vi "Keithley2400series_Start.vi"(4 "Serial Configuration":T1={"Baud Rate"=9600, "Parity"=0, "Data Bits"=8, "Stop Bits"=10, "Flow Control"=0} {"Flow Control" items=["None", "XON/XOFF", "RTS/CTS", "XON/XOFF & RTS/CTS", "DTR/DSR", "XON/XOFF & DTR/DSR"]; "Stop Bits" items=["1.0"=10, "1.5"=15, "2.0"=20]; "Data Bits" items=["7"=7, "8"=8]; "Parity" items=["None", "Odd", "Even", "Mark", "Space"]; "Baud Rate" items=["300"=300, "600"=600, "1200"=1200, "2400"=2400, "4800"=4800, "9600"=9600, "19200"=19200]}, 5 "Source Mode  (0: Voltage) 2":u16(ring) items=["Voltage", "Current"], 6 "Ограничение":dbl format="%.2f", 7 "Выход":dbl, 8 "VISA resource name":refnum<visa-resource-name>) -> (0 "error out":errorcluster, 1 "MEAS:Out":string, 2 "MEAS mode 0,Volt":dbl, 3 "VISA resource name out":refnum<visa-resource-name>)   [LabVIEW 2014]
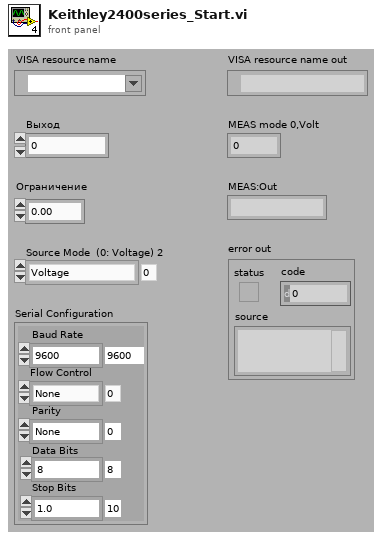
[diagram p1: front panel]
types:
  T1 = cluster{"Baud Rate":u32, "Parity":u16, "Data Bits":u16, "Stop Bits":u16, "Flow Control":u16}
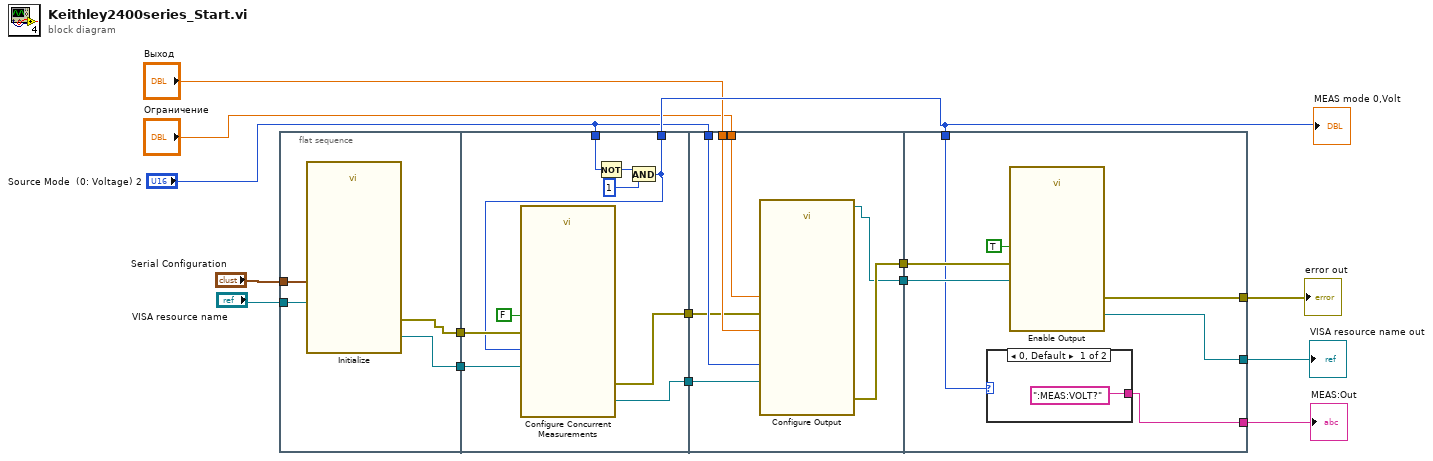
[diagram p0: block diagram]
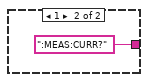
[diagram p2: hidden frame]
diagram:
  n1 = flat-sequence {
    tunnel: "VISA resource name" -> [w19]
    tunnel: "Serial Configuration" -> [w18]
    tunnel: [w17] -> w15
    tunnel: [w16] -> w14
    tunnel: "Source Mode  (0: Voltage) 2" -> [w25]
    tunnel: [w24] -> w13
    tunnel: [w23] -> w12
    tunnel: w15 -> [w22]
    tunnel: w14 -> [w21]
    tunnel: [w20] -> w9
    tunnel: "Ограничение" -> [w35]
    tunnel: "Выход" -> [w34]
    tunnel: "Source Mode  (0: Voltage) 2" -> [w33]
    tunnel: [w32] -> w11
    tunnel: [w31] -> w10
    tunnel: w13 -> [w30]
    tunnel: w12 -> [w29]
    tunnel: w11 -> [w41]
    tunnel: w10 -> [w40]
    tunnel: w9 -> [w39]
    tunnel: [w38] -> w5
    tunnel: [w37] -> w6
    tunnel: [w36] -> w7
    frame #0 {
      n2 = call "Initialize.vi"("Serial Configuration"=w18, "VISA resource name"=w19) -> ("error out"=w16:errorcluster, "VISA resource name out"=w17:refnum<visa-resource-name>)  [unwired: 8 in]
    }
    frame #1 {
      n3 = Not(x=w25) -> (.not. x?=w27:u16)
      n4 = And(x=w27, y=u16 1) -> (x .and. y?=w20:u16)
      n5 = call "Configure Concurrent Measurements.vi"("error in (no error)"=w21, "Measurement Selection (3: Volts, Current)"=w20, "Enable Concurrent Measurements (F: Disable)"=FALSE, "VISA resource name"=w22) -> ("error out"=w23:errorcluster, "VISA resource name out"=w24:refnum<visa-resource-name>)  [unwired: 6 in]
    }
    frame #2 {
      n6 = call "Configure Output.vi"("Source Mode  (0: Voltage)"=w33, "error in (no error)"=w29, "Compliance  Level (0.1)"=w35, "Output Level (0)"=w34, "VISA resource name"=w30) -> ("error out"=w32:errorcluster, "VISA resource name out"=w31:refnum<visa-resource-name>)  [unwired: 5 in]
    }
    frame #3 {
      n7 = case shown="0, Default" w39 {
        tunnel: [":MEAS:VOLT?" ":MEAS:CURR?"] -> w36
        frame 0, Default {
        }
        frame 1 {
        }
      }
      n8 = call "Enable Output.vi"("error in (no error)"=w41, "Enable Output (T: Enable)"=TRUE, "VISA resource name"=w40) -> ("error out"=w38:errorcluster, "VISA resource name out"=w37:refnum<visa-resource-name>)  [unwired: 7 in]
    }
  }
  "error out" <- w5
  "VISA resource name out" <- w6
  "MEAS:Out" <- w7
  "MEAS mode 0,Volt" <- w9
